vi "WeighContainer.vi"() -> (2 "Weight minus Baseline":dbl, 3 "Type":string)   [LabVIEW 2016, in "LEGO-PMR.lvrbt"]
uses:
  LEGO-PMR.lvrbt
  <vilib>/NXT/HiTechnic/HiTechnic Controls/HiTechnic Port.ctl
  <vilib>/NXT/Block Support/NXT_InputPort.ctl
  <vilib>/NXT/HiTechnic/HiTechnic Read/HiTechnic EOPD Sensor Long.vi
  <vilib>/NXT/Dual Mode Library/Waits/Wait_Num.vi
panel:
  out "Weight":dbl
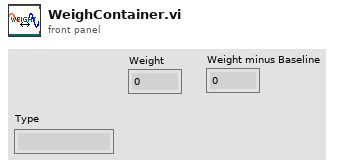
[diagram p1: front panel]
types:
  T1 = typedef "HiTechnic Port.ctl" = cluster{"Port":T2, "MUX Port":u8}
  T2 = typedef "NXT_InputPort.ctl" = u32
  T3 = typedef "LVHSConnector.ctl" = refnum<class "BrickReference.lvclass">
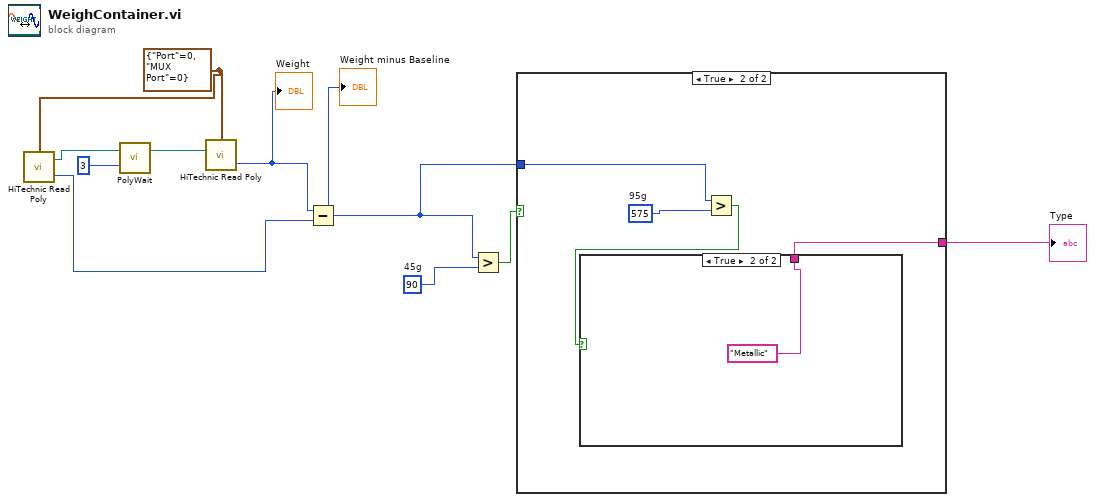
[diagram p0: block diagram]
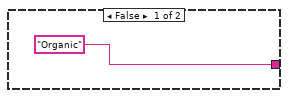
[diagram p2: hidden frame]
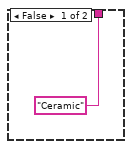
[diagram p3: hidden frame]
diagram:
  w2 = T1 {"Port"=0, "MUX Port"=0} ("Port/MUX")
  w7 = 90  # 45g
  n1 = call-poly <vilib>:"HiTechnic Read Poly.vi"("Port/MUX"=w2) -> ("EOPD Value"=w1:i16, "NXT/EV3"=w3:T3)  [unwired: 2 in]
  n2 = call-poly <vilib>:"PolyWait.vi"("Time (1 sec)"=3, "NXT/EV3"=w3) -> ("NXT/EV3"=w5:T3)  [unwired: 2 in]
  n3 = call-poly <vilib>:"HiTechnic Read Poly.vi"("NXT/EV3"=w5, "Port/MUX"=w2) -> ("EOPD Value"=w9:i16)  [unwired: 1 in, 1 out]
  "Weight" <- w9
  n4 = Subtract(x=w9, y=w1) -> (x-y=w10:i16)
  "Weight minus Baseline" <- w10
  n5 = Greater?(x=w10, y=w7) -> (0:w8:bool)
  n6 = case shown="True" w8 {
    tunnel: ["Organic" w12] -> w6
    tunnel: w10 -> [_ w14]
    frame False {
    }
    frame True {
      w15 = 575  # 95g
      n7 = Greater?(x=w14, y=w15) -> (0:w13:bool)
      n8 = case shown="True" w13 {
        tunnel: ["Ceramic" "Metallic"] -> w12
        frame False {
        }
        frame True {
        }
      }
    }
  }
  "Type" <- w6
